vi "get_reason_phrase_from_status_code.vi"(10 "status_code":u16) -> (1 "found?":bool, 2 "reason_phrase":string)   [LabVIEW 2020, in "HTTP Client reqwest.lvclass"]
uses:
  HTTP Client reqwest.lvclass
  HTTP Client reqwest.lvclass/HTTP Client reqwest.ctl
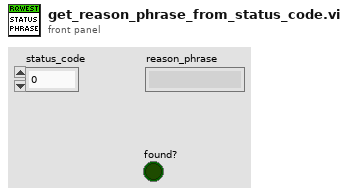
[diagram p1: front panel]
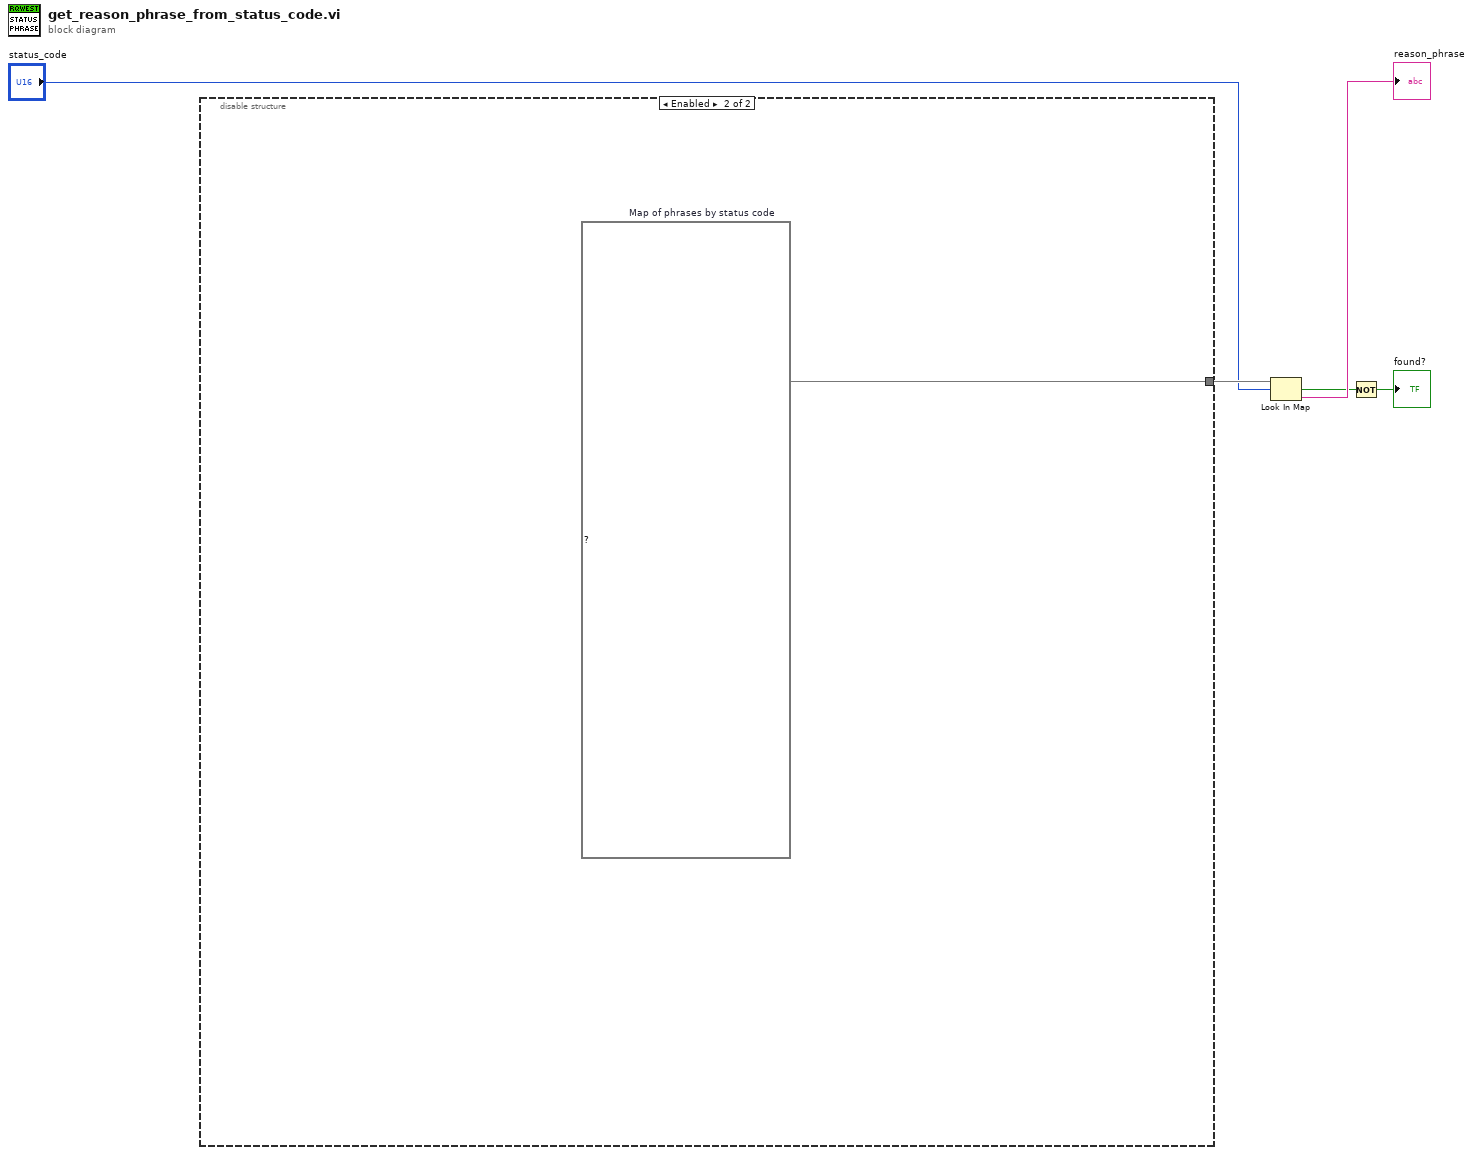
[diagram p0: block diagram]
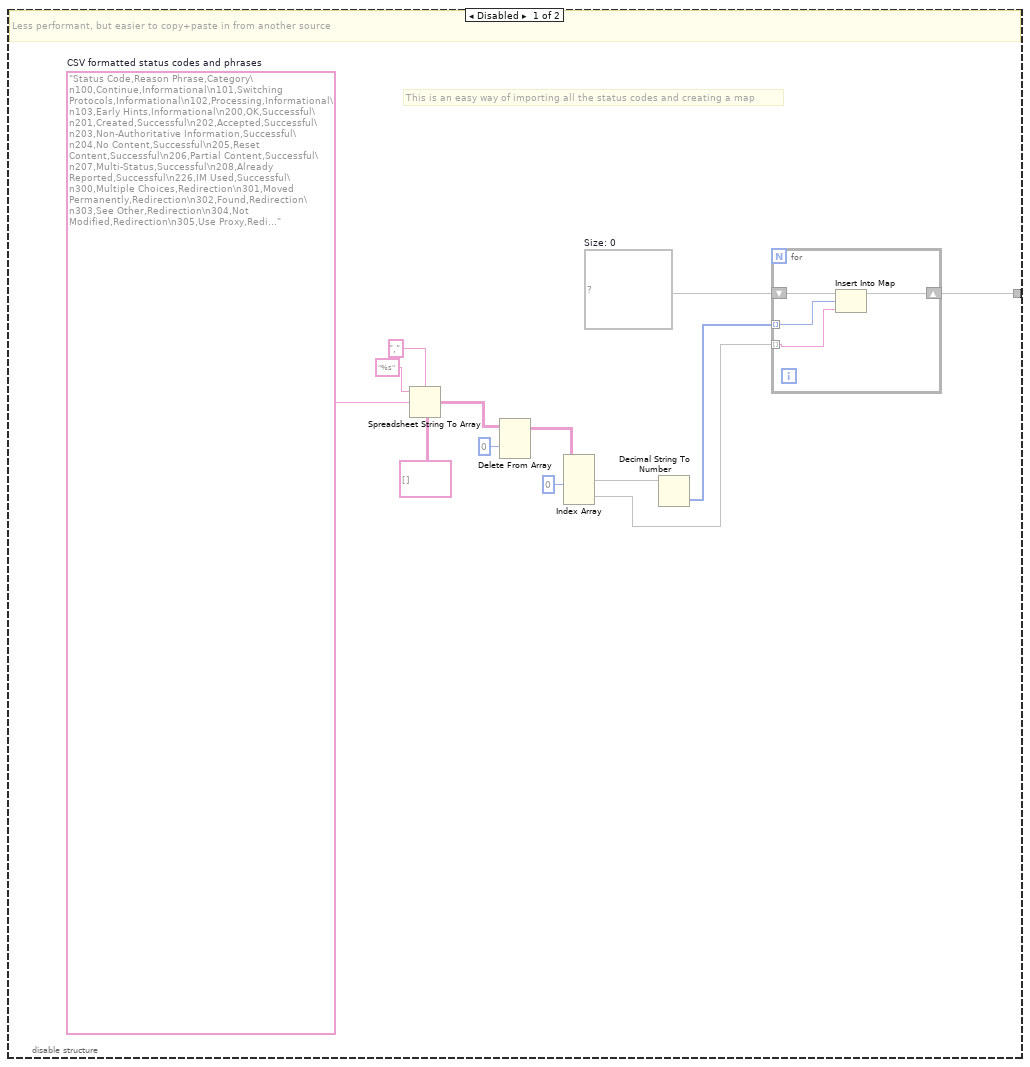
[diagram p2: hidden frame]
diagram:
  n1 = disable-structure shown="Enabled" {
    disable-tunnel: [w6 w23] -> w5
    frame Disabled {
      w9 = map{i32, string} {}  # Size: 0
      w18 = "Status Code,Reason Phrase,Category\n100,Continue,Informational\n101,Switching Protocols,Informational\n102,Processing,Informational\n103,Early Hints,Informational\n200,OK,Successful\n201,Created,Successful\n202,Accepted,Successful\n203,Non-Authoritative Information,Successful\n204,No Content,Successful\n205,Reset Content,Successful\n206,Partial Content,Successful\n207,Multi-Status,Successful\n208,Already Reported,Successful\n226,IM Used,Successful\n300,Multiple Choices,Redirection\n301,Moved Permanently,Redirection\n302,Found,Redirection\n303,See Other,Redirection\n304,Not Modified,Redirection\n305,Use Proxy,Redirection\n306,Unused,Redirection\n307,Temporary Redirect,Redirection\n308,Permanent Redirect,Redirection\n400,Bad Request,Client Error\n401,Unauthorized,Client Error\n402,Payment Required,Client Error\n403,Forbidden,Client Error\n404,Not Found,Client Error\n405,Method Not Allowed,Client Error\n406,Not Acceptable,Client Error\n407,Proxy Authentication Required,Client Error\n408,Request Timeout,Client Error\n409,Conflict,Client Error\n410,Gone,Client Error\n411,Length Required,Client Error\n412,Precondition Failed,Client Error\n413,Content Too Large,Client Error\n414,URI Too Long,Client Error\n415,Unsupported Media Type,Client Error\n416,Range Not Satisfiable,Client Error\n417,Expectation Failed,Client Error\n418,I'm a teapot,Client Error\n421,Misdirected Request,Client Error\n422,Unprocessable Content,Client Error\n423,Locked,Client Error\n424,Failed Dependency,Client Error\n425,Too Early,Client Error\n426,Upgrade Required,Client Error\n428,Precondition Required,Client Error\n429,Too Many Requests,Client Error\n431,Request Header Fields Too Large,Client Error\n451,Unavailable For Legal Reasons,Client Error\n500,Internal Server Error,Server Error\n501,Not Implemented,Server Error\n502,Bad Gateway,Server Error\n503,Service Unavailable,Server Error\n504,Gateway Timeout,Server Error\n505,HTTP Version Not Supported,Server Error\n506,Variant Also Negotiates,Server Error\n507,Insufficient Storage,Server Error\n508,Loop Detected,Server Error\n510,Not Extended,Server Error\n511,Network Authentication Required,Server Error"  # CSV formatted status codes and phrases
      # "This is an easy way of importing all the status codes and creating a map"
      # "Less performant, but easier to copy+paste in from another source"
      n2 = Spreadsheet String To Array(delimiter (Tab)=",", format string="%s", spreadsheet string=w18, array type (2D Dbl)=string[][] []) -> (array=w14:string[][])
      n3 = Delete From Array(array=w14, index (row)=0) -> (array with subset deleted=w12:string[][])  [unwired: 2 in, 1 out]
      n4 = Index Array(array=w12, index (col) #1=0 ("disabled index (col)")) -> (element #1=w10:string[], element #2=w7:string[])  [unwired: 3 in]
      n5 = Decimal String To Number(string=w10) -> (number=w8:i32[])  [unwired: 2 in, 1 out]
      n6 = for {
        shift-right: [w21] -> w6
        shift-left: w9 -> [w22]
        tunnel: w8 -> [w20] mode=indexing
        tunnel: w7 -> [w19] mode=indexing
        n7 = Insert Into Map(map in=w22, key=w20, value=w19) -> (map out=w21:map{i32, string})  [unwired: 2 out]
      }
    }
    frame Enabled {
      w23 = map{i32, string} {100="Continue", 101="Switching Protocols", 102="Processing", 103="Early Hints", 200="OK", 201="Created", 202="Accepted", 203="Non-Authoritative Information", 204="No Content", 205="Reset Content", 206="Partial Content", 207="Multi-Status", 208="Already Reported", 226="IM Used", 300="Multiple Choices", 301="Moved Permanently", 302="Found", 303="See Other", 304="Not Modified", 305="Use Proxy", 306="Unused", 307="Temporary Redirect", 308="Permanent Redirect", 400="Bad Request", 401="Unauthorized", 402="Payment Required", 403="Forbidden", 404="Not Found", 405="Method Not Allowed", 406="Not Acceptable", 407="Proxy Authentication Required", 408="Request Timeout", 409="Conflict", 410="Gone", 411="Length Required", 412="Precondition Failed", 413="Content Too Large", 414="URI Too Long", 415="Unsupported Media Type", 416="Range Not Satisfiable", 417="Expectation Failed", 418="I'm a teapot", 421="Misdirected Request", 422="Unprocessable Content", 423="Locked", 424="Failed Dependency", 425="Too Early", 426="Upgrade Required", 428="Precondition Required", 429="Too Many Requests", 431="Request Header Fields Too Large", 451="Unavailable For Legal Reasons", 500="Internal Server Error", 501="Not Implemented", 502="Bad Gateway", 503="Service Unavailable", 504="Gateway Timeout", 505="HTTP Version Not Supported", 506="Variant Also Negotiates", 507="Insufficient Storage", 508="Loop Detected", 510="Not Extended", 511="Network Authentication Required"}  # Map of phrases by status code
    }
  }
  n8 = Look In Map(map=w5, key="status_code") -> (key not found?=w2:bool, value=→"reason_phrase":string)  [unwired: 1 in]
  n9 = Not(x=w2) -> (.not. x?=→"found?":bool)
